vi "AIT 1553 - Parse Sysdef.vi"(0 "Device Reference in":T1 format="%.0x", 1 "Bus Config Info":T3, 5 "error in (no error)":errorcluster, 7 "FIFO Idx Qs":T5, 9 "Bus Page Ref":T1 format="%.0x") -> (8 "HWIn BaseRate BM":i32, 10 "HWIn BaseRate":i32, 12 "HWOut BaseRate":i32, 14 "Device Reference out":T1 format="%.0x", 15 "HWOutput Section Data":T6[](array[typedef]) {"Message Settings"."Driver Data"."First Word" min=8 max=31; "Message Settings"."Driver Data"."Num Bits" min=1 max=32; "Message Settings"."Driver Data"."Start Bit" min=8 max=31; "Message Settings"."Block Data Refs"."Data Reference" format="%.0x"}, 16 "HWInput Section Data":T6[](array[typedef]) {"Message Settings"."Driver Data"."First Word" min=8 max=31; "Message Settings"."Driver Data"."Num Bits" min=1 max=32; "Message Settings"."Driver Data"."Start Bit" min=8 max=31; "Message Settings"."Block Data Refs"."Data Reference" format="%.0x"}, 17 "output cluster":T2, 18 "Bus Controller Page Acyclic Frame Refs out":T1[](array[typedef]) format="%.0x", 19 "error out":errorcluster)   [LabVIEW 2013, in "AIT 1553 Custom Device.lvlib"]
uses:
  AIT 1553 Custom Device.lvlib
  RT Controls/AIT 1553 - RT HW Channel.ctl
  RT Controls/AIT 1553 - Bus Section.ctl
  RT Controls/AIT 1553 - RT Message Settings.ctl
  <vilib>/NI Veristand/Custom Device API/Block Data Reference.ctl
  <vilib>/NI Veristand/Custom Device API/Data Reference.ctl
  RT Controls/AIT 1553 - Driver Data.ctl
  Controls and Global/Start Bit.ctl
  Controls and Global/Number of Bits.ctl
  <vilib>/NI Veristand/Custom Device API/Custom Device Item Ref.ctl
  RT Controls/FIFO Idx Qs.ctl
  RT Controls/AIT 1553 - Board Config Info.ctl
  RT Controls/AIT 1553 - Hardware Type.ctl
  RT Controls/FIFO.ctl
  <vilib>/NI Veristand/Custom Device Tools/Custom Device Utility Library/RT Debug String Color Spec.ctl
  Controls and Global/Global.vi
  <vilib>/NI Veristand/Custom Device API/Custom Device API.lvlib
  <vilib>/NI Veristand/Custom Device Tools/Custom Device Utility Library/Custom Device Utility Library.lvlib
panel:
  # "BC"
  # "BM"
  # "RT"
  # "Bus - BC - Channel"
  # "Separate into Tx and Rx\nRx = Receive from HW\nTX = Transmit to HW"
  # "Message 1\n     Parameter 1\n     Parameter\n     .\n     .\n     Parameter n\nMessage 2\n     Parameter 1\n     Parameter\n     .\n     .\n     Parameter n"
  # "ARINC Bus"
  # "Channel 1\n     Label 1\n     Label\n     .\n     .\n     Label n\nChannel 2\n     Label 1\n     Label\n     .\n     .\n     Label n"
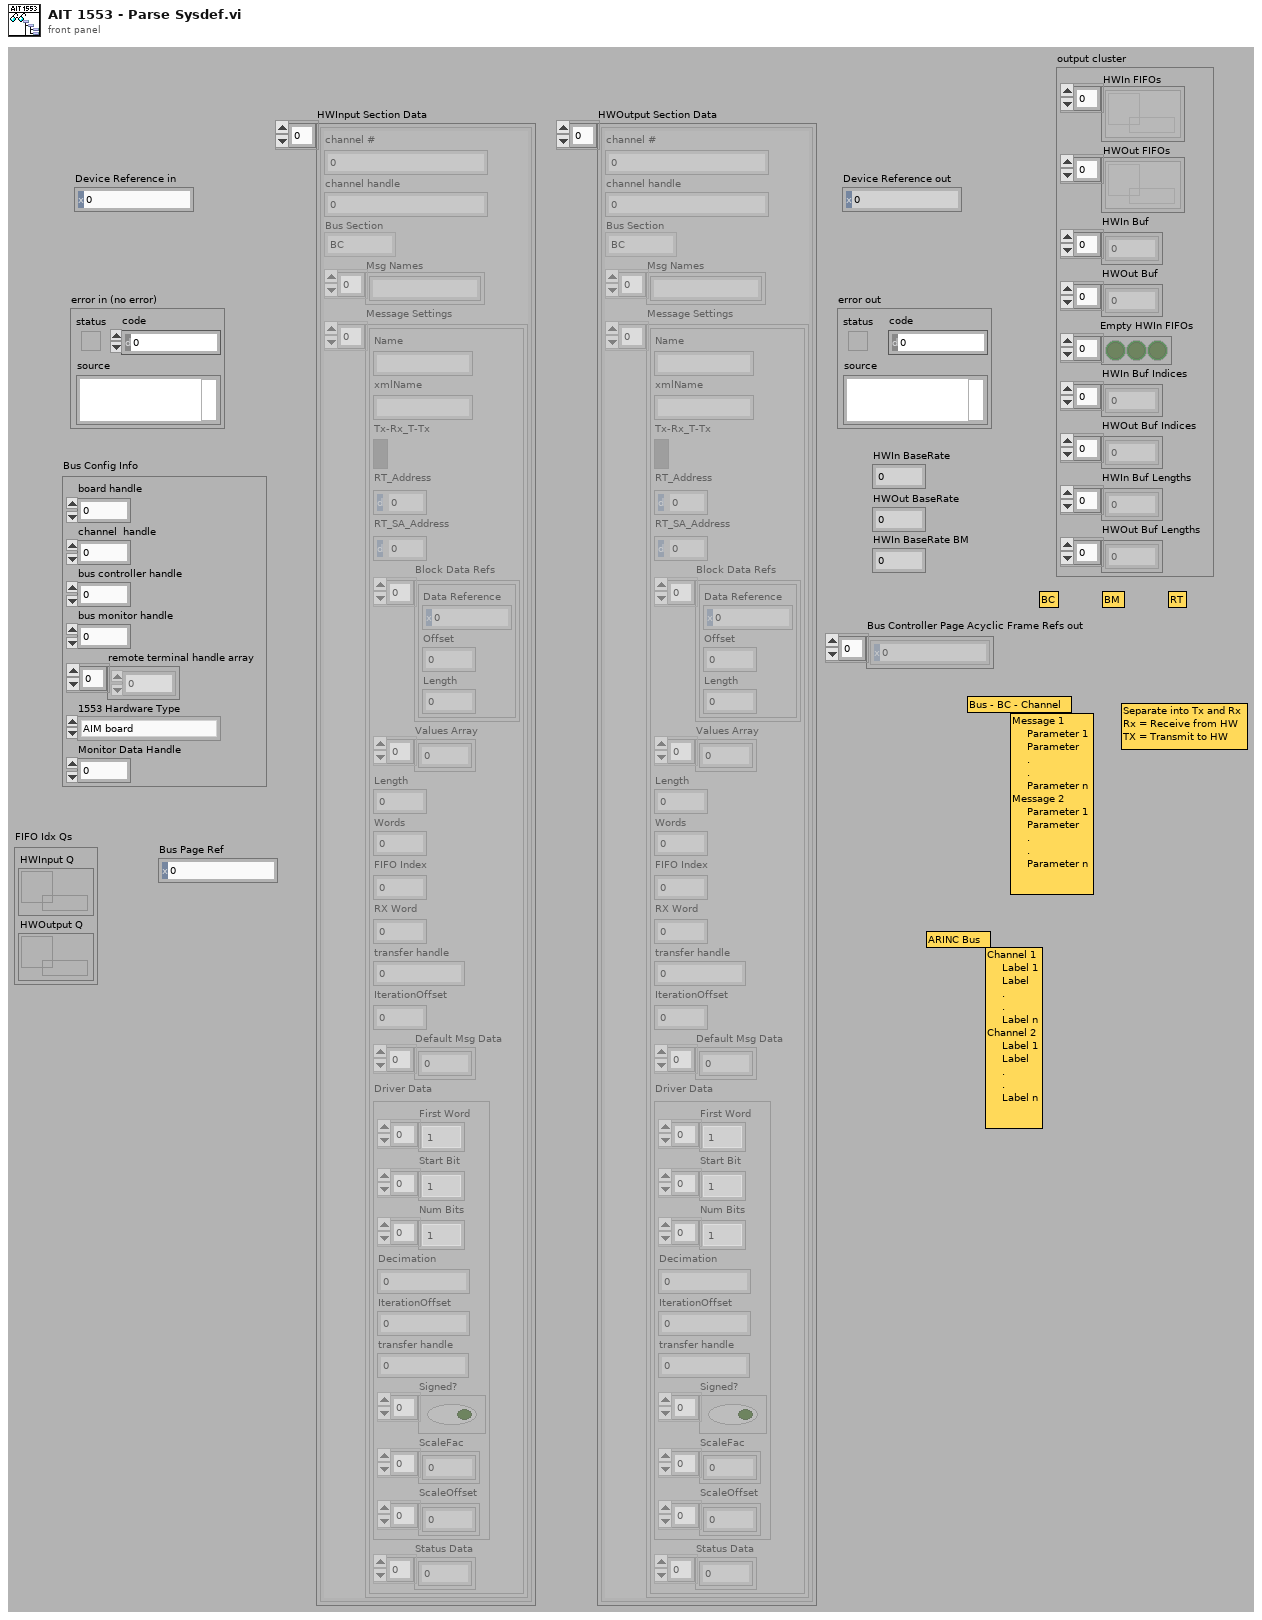
[diagram p1: front panel]
types:
  T1 = typedef "Custom Device API.lvlib/Custom Device Item Ref.ctl" = u64
  T2 = typedef "AIT 1553 Custom Device.lvlib/FIFO.ctl" = cluster{"HWIn FIFOs":refnum<k33>[], "HWOut FIFOs":refnum<k33>[], "HWIn Buf":dbl[], "HWOut Buf":dbl[], "Empty HWIn FIFOs":bool[], "HWIn Buf Indices":i32[], "HWOut Buf Indices":i32[], "HWIn Buf Lengths":i32[], "HWOut Buf Lengths":i32[]}
  T3 = typedef "AIT 1553 Custom Device.lvlib/AIT 1553 - Board Config Info.ctl" = cluster{"board handle":u32, "channel  handle":u32, "bus controller handle":u32, "bus monitor handle":u32, "remote terminal handle array":u32[], "1553 Hardware Type":T4, "Monitor Data Handle":u32}
  T4 = typedef "AIT 1553 Custom Device.lvlib/AIT 1553 - Hardware Type.ctl" = enum16{"AIM board", "AIT Board"}
  T5 = typedef "AIT 1553 Custom Device.lvlib/FIFO Idx Qs.ctl" = cluster{"HWInput Q":refnum<queue>, "HWOutput Q":refnum<queue>}
  T6 = typedef "AIT 1553 Custom Device.lvlib/AIT 1553 - RT HW Channel.ctl" = cluster{"channel #":u16, "channel handle":u32, "Bus Section":T7, "Msg Names":string[], "Message Settings":T8[]}
  T7 = typedef "AIT 1553 Custom Device.lvlib/AIT 1553 - Bus Section.ctl" = enum16{"BC", "BM", "RT"}
  T8 = typedef "AIT 1553 Custom Device.lvlib/AIT 1553 - RT Message Settings.ctl" = cluster{"Name":string, "xmlName":string, "Tx-Rx_T-Tx":bool, "RT_Address":u8, "RT_SA_Address":u8, "Block Data Refs":T9[], "Values Array":dbl[], "Length":i32, "Words":i32, "FIFO Index":i32, "RX Word":u32, "transfer handle":u32, "IterationOffset":i32, "Default Msg Data":u16[], "Driver Data":T11, "Status Data":u32[]}
  T9 = typedef "Custom Device API.lvlib/Block Data Reference.ctl" = cluster{"Data Reference":T10, "Offset":i32, "Length":i32}
  T10 = typedef "Custom Device API.lvlib/Data Reference.ctl" = i32
  T11 = typedef "AIT 1553 Custom Device.lvlib/AIT 1553 - Driver Data.ctl" = cluster{"First Word":T12[], "Start Bit":T12[], "Num Bits":T13[], "Decimation":i32, "IterationOffset":i32, "transfer handle":u32, "Signed?":bool[], "ScaleFac":dbl[], "ScaleOffset":dbl[]}
  T12 = typedef "AIT 1553 Custom Device.lvlib/Start Bit.ctl" = i32
  T13 = typedef "AIT 1553 Custom Device.lvlib/Number of Bits.ctl" = i32
  T14 = typedef "Custom Device Utility Library.lvlib/RT Debug String Color Spec.ctl" = u16
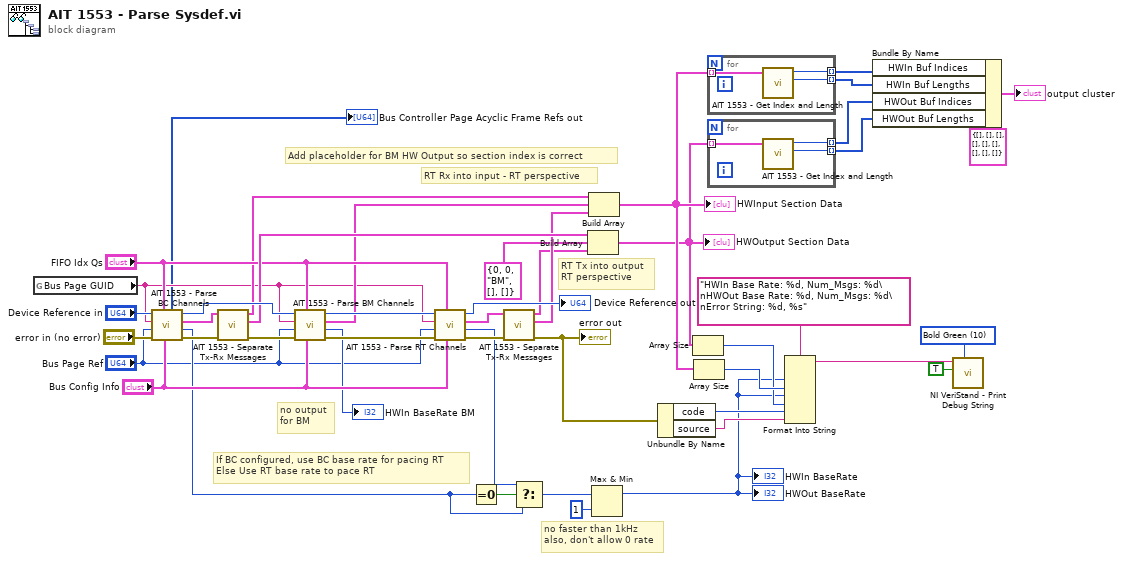
[diagram p0: block diagram]
diagram:
  w3 = T14 10 items=["Plain White"=7, "Bold White"=15, "Bold Blue"=9, "Bold Green"=10, "Bold Red"=12] ("Attribute")
  # "If BC configured, use BC base rate for pacing RT\nElse Use RT base rate to pace RT"
  # "no faster than 1kHz\nalso, don't allow 0 rate"
  # "Add placeholder for BM HW Output so section index is correct"
  # "RT Rx into input - RT perspective"
  # "RT Tx into output\nRT perspective"
  # "no output\nfor BM"
  n1 = global read "Global.vi" "Bus Page GUID"() -> (w13:string)
  n2 = call "AIT 1553 - Parse BC Channels.vi"("Bus Config Info"="Bus Config Info", "FIFO Idx Qs"="FIFO Idx Qs", "error in (no error)"="error in (no error)", "Bus Page Ref"="Bus Page Ref", "Section GUID"=w13, "Device Reference in"="Device Reference in") -> ("error out"=w38:errorcluster, "Section BaseRate"=w7:u32, "HW Channel - BC Section"=w36:T6, "Device Reference out"=w39:T1, "Bus Controller Page Acyclic Frame Refs out"=→"Bus Controller Page Acyclic Frame Refs out":T1[])  [unwired: 1 in]
  n3 = call "AIT 1553 - Separate Tx-Rx Messages.vi"("error in (no error)"=w38, "HW Channel - Section in"=w36) -> ("error out"=w37:errorcluster, "HW Channel Rx - Section out"=w35:T6, "HW Channel Tx - Section out"=w23:T6)  [unwired: 7 in]
  n4 = call "AIT 1553 - Parse BM Channels.vi"("Bus Config Info"="Bus Config Info", "FIFO Idx Qs"="FIFO Idx Qs", "error in (no error)"=w37, "Bus Page Ref"="Bus Page Ref", "Section GUID"=w13, "Device Reference in"=w39) -> ("error out"=w29:errorcluster, "Section BaseRate"=→"HWIn BaseRate BM":u32, "HW Channel - BM Section"=w27:T6, "Device Reference out"=w28:T1)  [unwired: 2 in]
  n5 = call "AIT 1553 - Parse RT Channels.vi"("Bus Config Info"="Bus Config Info", "FIFO Idx Qs"="FIFO Idx Qs", "error in (no error)"=w29, "Bus Page Ref"="Bus Page Ref", "Section GUID"=w13, "Device Reference in"=w28) -> ("error out"=w33:errorcluster, "Section BaseRate"=w9:u32, "HW Channel - RT Section"=w31:T6, "Device Reference out"=→"Device Reference out":T1)  [unwired: 2 in]
  n6 = Equal To 0?(x=w7) -> (x = 0?=w10:bool)
  n7 = call "AIT 1553 - Separate Tx-Rx Messages.vi"("error in (no error)"=w33, "HW Channel - Section in"=w31) -> ("error out"=w14:errorcluster, "HW Channel Rx - Section out"=w26:T6, "HW Channel Tx - Section out"=w25:T6)  [unwired: 7 in]
  "error out" <- w14
  n8 = Select(t=w9, s=w10, f=w7) -> (s? t:f=w6:u32)
  n9 = Build Array(w35, T6 {"channel #"=0, "channel handle"=0, "Bus Section"=enum."BM", "Msg Names"=[], "Message Settings"=[]} ("element"), w25) -> (w21:T6[])
  "HWOutput Section Data" <- w21
  n10 = Build Array(w23, w27, w26) -> (w22:T6[])
  "HWInput Section Data" <- w22
  n11 = Max & Min(x=w6, y=u32 1) -> (max(x,y)=w1:u32)  [unwired: 1 out]
  "HWIn BaseRate" <- w1
  "HWOut BaseRate" <- w1
  n12 = Unbundle By Name(w14) -> ("code"=w44:i32, "source"=w43:string)
  n13 = Array Size(array=w21) -> (size(s)=w40:i32)
  n14 = Array Size(array=w22) -> (size(s)=w41:i32)
  n15 = for {
    tunnel: w22 -> [w49] mode=indexing
    tunnel: [w48] -> w19 mode=indexing
    tunnel: [w47] -> w18 mode=indexing
    n16 = call "AIT 1553 - Get Index and Length.vi"("Section"=w49) -> ("Length"=w47:i32, "FIFO Index"=w48:i32)  [unwired: 9 in]
  }
  n17 = for {
    tunnel: w21 -> [w52] mode=indexing
    tunnel: [w51] -> w17 mode=indexing
    tunnel: [w50] -> w16 mode=indexing
    n18 = call "AIT 1553 - Get Index and Length.vi"("Section"=w52) -> ("Length"=w50:i32, "FIFO Index"=w51:i32)  [unwired: 9 in]
  }
  n19 = Format Into String(format string="HWIn Base Rate: %d, Num_Msgs: %d\nHWOut Base Rate: %d, Num_Msgs: %d\nError String: %d, %s", w1, w41, w1, w40, w44, w43) -> (resulting string=w5:string)  [unwired: 2 in, 1 out]
  n20 = Bundle By Name(cluster=T2 {"HWIn FIFOs"=[], "HWOut FIFOs"=[], "HWIn Buf"=[], "HWOut Buf"=[], "Empty HWIn FIFOs"=[], "HWIn Buf Indices"=[], "HWOut Buf Indices"=[], "HWIn Buf Lengths"=[], "HWOut Buf Lengths"=[]} ("output cluster"), "HWIn Buf Indices"=w19, "HWIn Buf Lengths"=w18, "HWOut Buf Indices"=w17, "HWOut Buf Lengths"=w16) -> (→"output cluster":T2)
  n21 = call <vilib>:"NI VeriStand - Print Debug String.vi"("Attribute"=w3, "Add to log file? (T)"=TRUE, "Message"=w5) -> ()  [unwired: 8 in, 1 out]
